vi "PCO_SetTransferParametersAuto.vi"(8 "error in (no error)":errorcluster {"code" format="%x"}, 11 "ph":u64) -> (0 "error out":errorcluster {"code" format="%x"}, 2 "ErrorMessage":i32 format="%x", 3 "ph out":u64)   [LabVIEW 2019, in "SDK.lvlib" / "SpecialCommandsEdge.lvlib"]
doc: "<b>Description:</b>\nThis function can be used to setup the correct transfer parameters for a pco.edge 5.5 with Camera Link interface, when used in Rolling Shutter or Global Reset mode. The SDK automatically selects appropriate parameters for the transfer. Depending on the current camera settings either PCO_CL_DATAFORMAT_5x16 or PCO_CL_DATAFORMAT_5x12L with the appropriate LUT is set. The current SCCMOS Readout Format remains as it is.\nPlease set buffer and ilen to zero. If a valid memory buffer is given as input, the current settings are returned as transfer parameter structure PCO_SC2_CL_TRANSFER_PARAM, but you have to set all buffer members to zero before calling.\n\n<b>Supported camera type</b>\npco.edge 5.5 with Camera Link interface\n\n<b>Descriptor dependency:</b>\nNone"
uses:
  SpecialCommandsEdge.lvlib
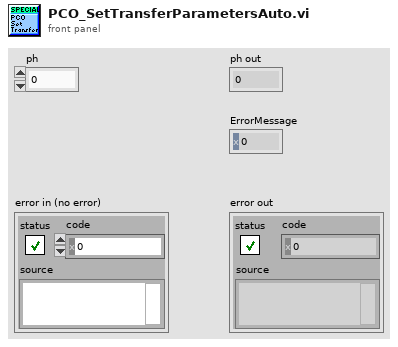
[diagram p1: front panel]
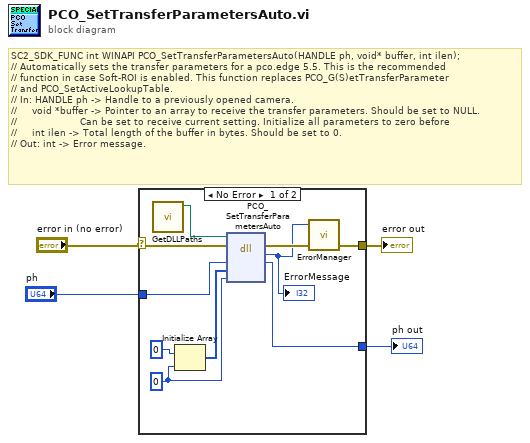
[diagram p0: block diagram]
diagram:
  # "SC2_SDK_FUNC int WINAPI PCO_SetTransferParametersAuto(HANDLE ph, void* buffer, int ilen);\n// Automatically sets the transfer parameters for a pco.edge 5.5. This is the recommended\n// function in case Soft-ROI is enabled. This function replaces PCO_G(S)etTransferParameter\n// and PCO_SetActiveLookupTable.\n// In: HANDLE ph -> Handle to a previously opened camera.\n//     void *buffer -> Pointer to an array to receive the transfer parameters. Should be set to NULL.\n//                     Can be set to receive current setting. Initialize all parameters to zero before\n//     int ilen -> Total length of the buffer in bytes. Should be set to 0.\n// Out: int -> Error message."
  n1 = case shown="No Error" "error in (no error)" {
    selector: "error in (no error)" -> [w9 w16]
    tunnel: "ph" -> [w14 w15]
    tunnel: [w13 w15] -> w3
    tunnel: [w7 w16] -> w2
    frame No Error {
      w10 = 0 ("ilen")
      n2 = call "GetDLLPaths.vi"() -> ("SC2_Cam_Path"=w5:path)  [unwired: 9 in, 2 out]
      n3 = Initialize Array(u32 0, w10) -> (w11:u32[])
      n4 = dll-call lib="?" fn="PCO_SetTransferParametersAuto"(path in=w5, error in=w9, "ph"=w14, "buffer"=w11, "ilen"=w10) -> (error out=w8:errorcluster, "return type"=w6:i32, "ph"=w13:u64)  [unwired: 3 in, 1 out]
      "ErrorMessage" <- w6
      n5 = call "ErrorManager.vi"("error in (no error)"=w8, "error code"=w6) -> ("error out"=w7:errorcluster)  [unwired: 3 in]
    }
    frame Error {
    }
  }
  "ph out" <- w3
  "error out" <- w2
